vi "Drive Modifications.vi"(1 "Mods In":T1) -> (0 "Mods Out":T2)   [LabVIEW 2016]
uses:
  Robot Global Data.vi
  <vilib>/Rock Robotics/Network Tables/NT Write Boolean.vi
  <vilib>/Rock Robotics/Network Tables/NT Write Number.vi
panel:
  out "dt":u32
  out "Robot Position":cluster{dbl[], dbl[]}[](graph)
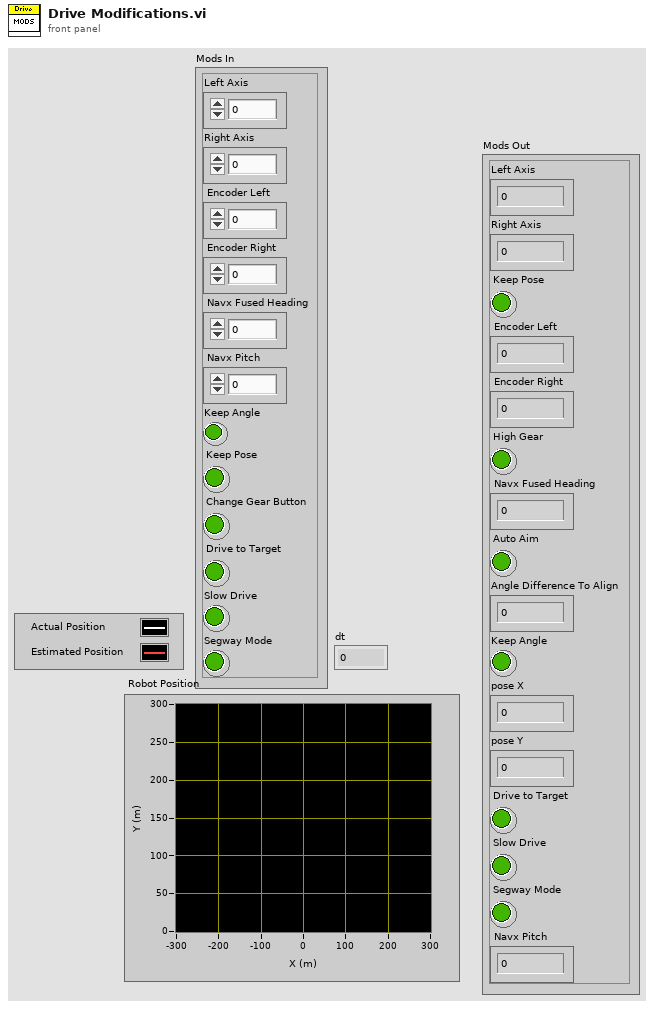
[diagram p1: front panel]
types:
  T1 = cluster{"Left Axis":dbl, "Right Axis":dbl, " Encoder Left":dbl, " Encoder Right":dbl, " Navx Fused Heading":dbl, " Navx Pitch":dbl, "Keep Angle":bool, "Keep Pose":bool, "Change Gear Button":bool, "Drive to Target":bool, "Slow Drive":bool, "Segway Mode":bool}
  T2 = cluster{"Left Axis":dbl, "Right Axis":dbl, "Keep Pose":bool, " Encoder Left":dbl, " Encoder Right":dbl, "High Gear":bool, " Navx Fused Heading":dbl, "Auto Aim":bool, "Angle Difference To Align":dbl, "Keep Angle":bool, "pose X":dbl, "pose Y":dbl, "Drive to Target":bool, "Slow Drive":bool, "Segway Mode":bool, " Navx Pitch":dbl}
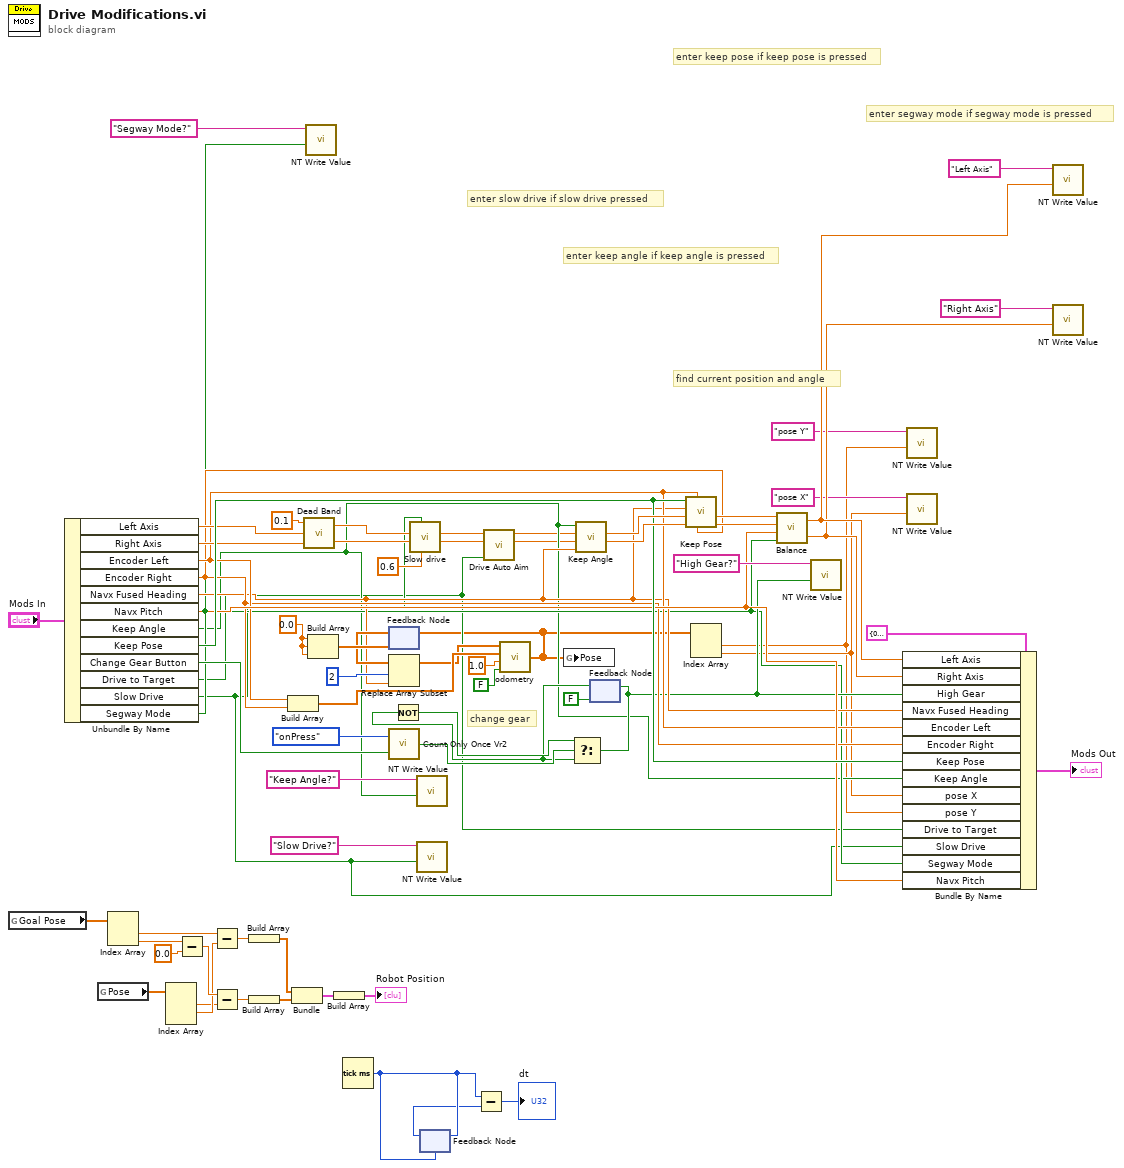
[diagram p0: block diagram]
diagram:
  w47 = 0.0 ("element")
  # "change gear"
  # "find current position and angle"
  # "enter segway mode if segway mode is pressed"
  # "enter keep pose if keep pose is pressed"
  # "enter keep angle if keep angle is pressed"
  # "enter slow drive if slow drive pressed"
  n1 = global read "Robot Global Data.vi" "Goal Pose"() -> (w4:dbl[])
  n2 = Unbundle By Name("Mods In") -> ("Left Axis"=w59:dbl, "Right Axis"=w58:dbl, "Encoder Left"=w51:dbl, "Encoder Right"=w50:dbl, "Navx Fused Heading"=w41:dbl, "Navx Pitch"=w52:dbl, "Keep Angle"=w30:bool, "Keep Pose"=w63:bool, "Change Gear Button"=w61:bool, "Drive to Target"=w25:bool, "Slow Drive"=w28:bool, "Segway Mode"=w32:bool)
  n3 = global read "Robot Global Data.vi" "Pose"() -> (w17:dbl[])
  n4 = Index Array(array=w4) -> (element #1=w6:dbl, element #2=w5:dbl)  [unwired: 2 in]
  n5 = Index Array(array=w17) -> (element #1=w13:dbl, element #2=w14:dbl)  [unwired: 3 in, 1 out]
  n6 = Subtract(x=w5, y=0.0) -> (x-y=w15:dbl)
  n7 = Subtract(x=w6, y=w14) -> (x-y=w8:dbl)
  n8 = Subtract(x=w15, y=w13) -> (x-y=w7:dbl)
  n9 = Build Array(w8) -> (w12:dbl[])
  n10 = Build Array(w7) -> (w11:dbl[])
  n11 = Build Array(w51, w50) -> (w49:dbl[])
  n12 = Bundle(w12, w11) -> (w10:cluster{dbl[], dbl[]})  [unwired: 1 in]
  n13 = call "Dead Band.vi"("Axis 2 In"=w58, "Axis 1 In"=w59, "Dead Band"=0.1) -> ("Axis 2 Out"=w57:dbl, "Axis 1 Out"=w56:dbl)
  n14 = call-poly <vilib>:"NT Write Value.vi"("Boolean"=w32, "Name"="Segway Mode?") -> ()  [unwired: 9 in, 1 out]
  n15 = Build Array(w47, w47, w47) -> (w48:dbl[])
  n16 = Build Array(w10) -> (→"Robot Position":cluster{dbl[], dbl[]}[])
  n17 = Tick Count (ms)() -> (millisecond timer value=w3:u32)
  n18 = feedback #1(w48) -> (w46:dbl[])
  n19 = Replace Array Subset(array=w46, new element=w41, index=2) -> (w43:dbl[])
  n20 = call "Count Only Once Vr2.vi"("InValue"=w61, "Action"=enum16{"onPress", "onRelease", "Both"}."onPress") -> ("Result"=w69:bool)
  n21 = call "Slow drive.vi"("Slow drive to"=0.6, "Slow?"=w28, "Y-Axis"=w57, "X-Axis"=w56) -> ("Y - Axis out"=w26:dbl, "X-Axis out"=w27:dbl)  [unwired: 6 in]
  n22 = call-poly <vilib>:"NT Write Value.vi"("Boolean"=w30, "Name"="Keep Angle?") -> ()  [unwired: 9 in, 1 out]
  n23 = call-poly <vilib>:"NT Write Value.vi"("Boolean"=w28, "Name"="Slow Drive?") -> ()  [unwired: 9 in, 1 out]
  n24 = feedback #2(w3) -> (w2:u32)
  n25 = feedback-in #2(w3) -> ()
  n26 = Subtract(x=w3, y=w2) -> (x-y=→"dt":u32)
  n27 = call "Drive Auto Aim.vi"("Auto Aim"=w25, "Right Axis 2"=w26, "Left Axis 2"=w27) -> ("Right Axis"=w23:dbl, "Left Axis"=w24:dbl)  [unwired: 7 in]
  n28 = call "odometry.vi"("reset"=FALSE, "distance between sides of wheels"=1.0, "encoders in"=w49, "state in"=w43) -> ("state out"=w18:dbl[])
  n29 = feedback-in #1(w18) -> ()
  n30 = global write "Robot Global Data.vi" "Pose"(w18) -> ()
  n31 = call "Keep Angle.vi"("Angle"=w41, "Right Speed"=w23, "Left Speed"=w24, "Keep Angle"=w30) -> ("Right"=w65:dbl, "Left"=w66:dbl)  [unwired: 6 in]
  n32 = feedback #3(FALSE) -> (w39:bool)
  n33 = Not(x=w39) -> (.not. x?=w40:bool)
  n34 = Select(t=w40, s=w69, f=w39) -> (s? t:f=w38:bool)
  n35 = feedback-in #3(w38) -> ()
  n36 = call "Keep Pose.vi"("Encoder Right"=w50, "Encoder Left"=w51, "Right Axis"=w65, "Left Axis"=w66, "Angle"=w41, "Keep Pose"=w63) -> ("Right"=w53:dbl, "Left"=w54:dbl)  [unwired: 4 in]
  n37 = Index Array(array=w18) -> (element #1=w19:dbl, element #2=w21:dbl)  [unwired: 2 in]
  n38 = call "Balance.vi"("Segway Mode?"=w32, "Pitch Angle"=w52, "Right Axis"=w53, "Left Axis"=w54) -> ("Right Axis"=w34:dbl, "Left Axis"=w36:dbl)
  n39 = call-poly <vilib>:"NT Write Value.vi"("Boolean"=w38, "Name"="High Gear?") -> ()  [unwired: 9 in, 1 out]
  n40 = Bundle By Name(cluster=T2 {"Left Axis"=0.0, "Right Axis"=0.0, "Keep Pose"=FALSE, " Encoder Left"=0.0, " Encoder Right"=0.0, "High Gear"=FALSE, " Navx Fused Heading"=0.0, "Auto Aim"=FALSE, "Angle Difference To Align"=0.0, "Keep Angle"=FALSE, "pose X"=0.0, "pose Y"=0.0, "Drive to Target"=FALSE, "Slow Drive"=FALSE, "Segway Mode"=FALSE, " Navx Pitch"=0.0} ("Mods Out 2"), "Left Axis"=w36, "Right Axis"=w34, "High Gear"=w38, "Navx Fused Heading"=w41, "Encoder Left"=w51, "Encoder Right"=w50, "Keep Pose"=w63, "Keep Angle"=w30, "pose X"=w21, "pose Y"=w19, "Drive to Target"=w25, "Slow Drive"=w28, "Segway Mode"=w32, "Navx Pitch"=w52) -> (→"Mods Out":T2)
  n41 = call-poly <vilib>:"NT Write Value.vi"("Numeric"=w19, "Name"="pose Y") -> ()  [unwired: 9 in, 1 out]
  n42 = call-poly <vilib>:"NT Write Value.vi"("Numeric"=w21, "Name"="pose X") -> ()  [unwired: 9 in, 1 out]
  n43 = call-poly <vilib>:"NT Write Value.vi"("Numeric"=w36, "Name"="Left Axis") -> ()  [unwired: 9 in, 1 out]
  n44 = call-poly <vilib>:"NT Write Value.vi"("Numeric"=w34, "Name"="Right Axis") -> ()  [unwired: 9 in, 1 out]
